vi "Ejercicio_21_Solid.vi"() -> ()   [LabVIEW 2020]
uses:
  <vilib>/Motion/Express/_s/nimc.ex.straightLineMove.startStraightLineMove.axis.modeAbsolute.0.vi
  <vilib>/Motion/BlockNode/FB.NIMotion.xnode
panel:
  in  "stop":bool
  in  "position":dbl=1000.0
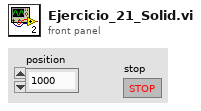
[diagram p1: front panel]
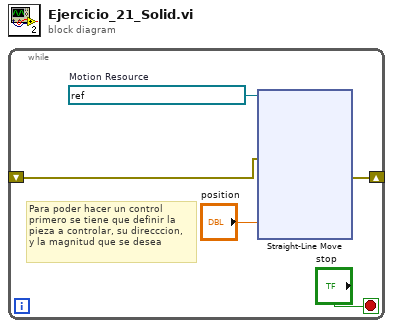
[diagram p0: block diagram]
diagram:
  n1 = while {
    shift-right: [w4] -> _
    shift-left: _ -> [w3]
    stop <- "stop" stop-if-true
    w2 = refnum<k21> "nism://My Computer/Axis 1"  # Motion Resource
    # "Para poder hacer un control\nprimero se tiene que definir la \npieza a controlar, su direcccion,\ny la magnitud que se desea"
    n2 = xnode ("Straight-Line Move")("position"="position", "resource"=w2, "error in"=w3) -> ("error out"=w4:errorcluster)  [unwired: 7 in, 2 out]
  }
